vi "Scale arcsec To deg.vi"(11 "arcsec":dbl) -> (3 "deg":dbl)   [LabVIEW 2015, in "Utility.lvlib"]
uses:
  Utility.lvlib
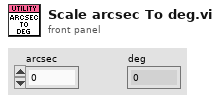
[diagram p1: front panel]
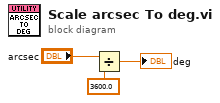
[diagram p0: block diagram]
diagram:
  n1 = Divide(x="arcsec", y=3600.0) -> (x/y=→"deg":dbl)
